vi "TWM Client Wait ACK.vi"(5 "timeout [ms] (3000)":i32=3000, 7 "key string":string="TWM:command:EndOfPacket", 8 "error in":errorcluster, 10 "command header":string, 11 "handle":i32) -> (0 "error out":errorcluster, 3 "handle out":i32)   [LabVIEW 2020, in "TWM Client.lvlib"]
doc: "Wait for ACK message from server."
uses:
  TWM Client.lvlib
  <vilib>/Utility/error.llb/Error Cluster From Error Code.vi
  Get 1D String.vi
  <vilib>/ErrorRing/Error Ring.xnode
  infolib.lvlib
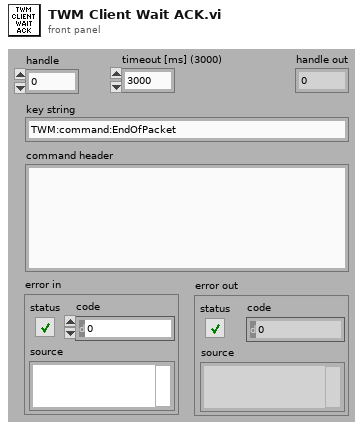
[diagram p1: front panel]
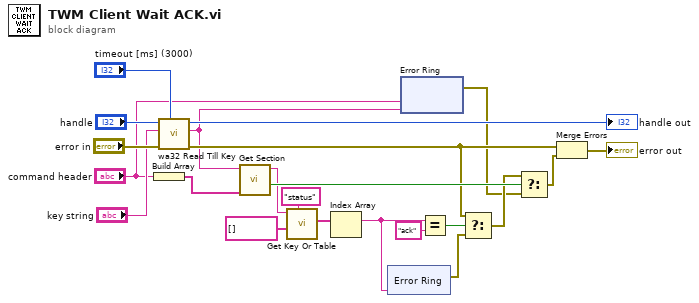
[diagram p0: block diagram]
diagram:
  n1 = Build Array("command header") -> (w3:string[])
  n2 = call "wa32 Read Till Key.vi"("timeout [ms] (1000)"="timeout [ms] (3000)", "error in"="error in", "key string"="key string", "handle"="handle") -> ("error out"=w12:errorcluster, "read message"=w2:string, "handle out"=→"handle out":i32)  [unwired: 5 in]
  n3 = call "Get Section.vi"("sections"=w3, "info data"=w2) -> ("exist"=w18:bool, "section part"=w17:string)  [unwired: 7 in, 1 out]
  n4 = call-poly "Get Key Or Table.vi"("key description"="status", "string"=string[] [], "info data"=w17) -> ("value"=w9:string[])  [unwired: 5 in, 3 out]
  n5 = Index Array(array=w9) -> (element=w5:string)  [unwired: 1 in]
  n6 = xnode "Error Ring"("parameter 0"=w5) -> ("error out"=w8:errorcluster)
  n7 = xnode "Error Ring"("parameter 0"="command header", "parameter 1"=w2) -> ("error out"=w7:errorcluster)
  n8 = Equal?(x=w5, y="ack") -> (x = y?=w14:bool)
  n9 = Select(t=w12, s=w14, f=w8) -> (s? t:f=w13:errorcluster)
  n10 = Select(t=w13, s=w18, f=w7) -> (s? t:f=w11:errorcluster)
  n11 = Merge Errors(w12, w11) -> (→"error out":errorcluster)
